vi "Save Message from Event Log.vi"(8 "error in (no error)":errorcluster, 9 "Event Type (0: Error)":u16(ring) items=["Error", "Warning", "Informational", "All"], 10 "File Name":string, 11 "VISA resource name":refnum<visa-resource-name>) -> (0 "error out":errorcluster, 3 "VISA resource name out":refnum<visa-resource-name>)   [LabVIEW 2020, in "Keithley 2450.lvlib"]
doc: "This saves the event log to a file on a USB flash drive."
uses:
  Keithley 2450.lvlib
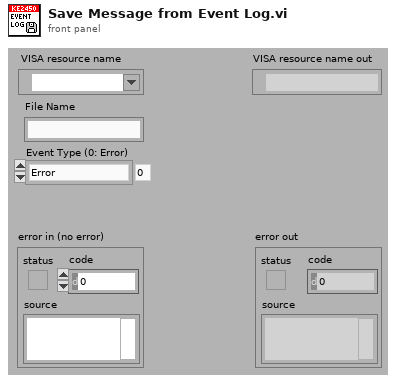
[diagram p1: front panel]
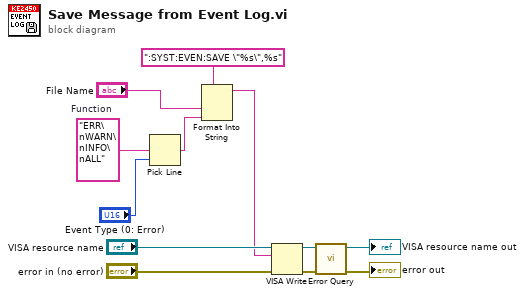
[diagram p0: block diagram]
diagram:
  w2 = "ERR\nWARN\nINFO\nALL"  # Function
  n1 = Pick Line(multi-line string=w2, line index="Event Type (0: Error)") -> (output string=w3:string)  [unwired: 1 out]
  n2 = Format Into String(format string=":SYST:EVEN:SAVE \"%s\",%s", "File Name", w3) -> (resulting string=w6:string)  [unwired: 2 in, 1 out]
  n3 = VISA Write(VISA resource name="VISA resource name", write buffer=w6, error in (no error)="error in (no error)") -> (VISA resource name out=w8:refnum<visa-resource-name>, error out=w7:errorcluster)  [unwired: 1 out]
  n4 = call "Error Query.vi"("error in (no error)"=w7, "VISA resource name"=w8) -> ("error out"=→"error out":errorcluster, "VISA resource name out"=→"VISA resource name out":refnum<visa-resource-name>)  [unwired: 8 out]
